vi "Self.vi"(9 "Is Priority":bool, 10 "Msg":refnum<class "Msg.lvclass">, 11 "jettl Actor in":refnum<class "jettl Actor.lvclass">) -> (3 "jettl Actor out":refnum<class "jettl Actor.lvclass">)   [LabVIEW 2021, in "jettl.lvlib" / "Temporary Actor.lvlib" / "jettl Actor.lvclass"]
uses:
  jettl Actor.lvclass
  Msg/Msg.lvclass
  Utilities/Relation.ctl
  jettl Actor.lvclass/jettl Actor.ctl
  Addresses Strategy/Addresses Strategy/Addresses Strategy.lvclass
  Sender/Sender/Sender.lvclass
  Utilities/Utilities.lvlib
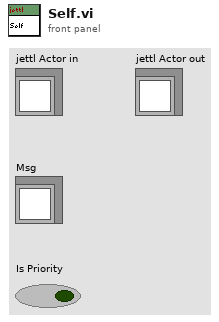
[diagram p1: front panel]
types:
  T1 = typedef "jettl.lvlib/Utilities.lvlib/Relation.ctl" = enum16{"Self", "Creator", "Created"}
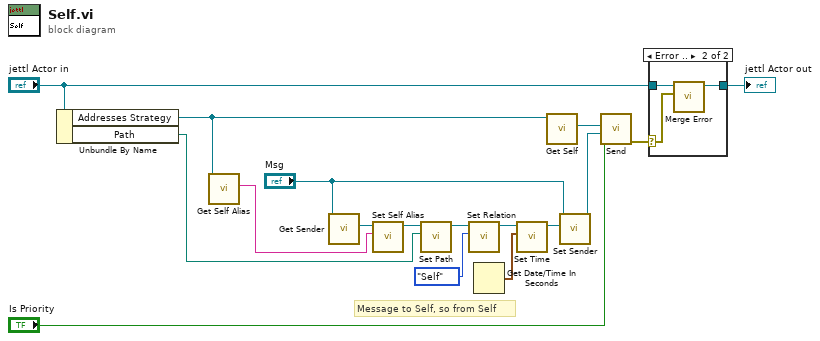
[diagram p0: block diagram]
diagram:
  # "Message to Self, so from Self"
  n1 = Unbundle By Name("jettl Actor in") -> ("Addresses Strategy"=w11:refnum<class "Addresses Strategy.lvclass">, "Path"=w1:path)
  n2 = call-dynamic "Get Self Alias.vi"("Addresses Strategy in"=w11) -> ("Self Alias"=w4:string)  [unwired: 10 in]
  n3 = call-dynamic "Get Sender.vi"("Msg in"="Msg") -> ("Sender"=w6:refnum<class "Sender.lvclass">)  [unwired: 10 in]
  n4 = call-dynamic "Set Self Alias.vi"("Self Alias"=w4, "Sender in"=w6) -> ("Sender out"=w9:refnum<class "Sender.lvclass">)  [unwired: 9 in]
  n5 = call-dynamic "Set Path.vi"("Path"=w1, "Sender in"=w9) -> ("Sender out"=w8:refnum<class "Sender.lvclass">)  [unwired: 9 in]
  n6 = call-dynamic "Set Relation.vi"("Relation"=Relation."Self", "Sender in"=w8) -> ("Sender out"=w7:refnum<class "Sender.lvclass">)  [unwired: 9 in]
  n7 = Get Date/Time In Seconds() -> (seconds since 1Jan1904=w2:timestamp)
  n8 = call-dynamic "Set Time.vi"("Time"=w2, "Sender in"=w7) -> ("Sender out"=w5:refnum<class "Sender.lvclass">)  [unwired: 9 in]
  n9 = call-dynamic "Get Self.vi"("Addresses Strategy in"=w11) -> ("Self"=w15:refnum<user-event>)  [unwired: 10 in]
  n10 = call-dynamic "Set Sender.vi"("Sender"=w5, "Msg in"="Msg") -> ("Msg out"=w12:refnum<class "Msg.lvclass">)  [unwired: 9 in]
  n11 = call "Send.vi"("Is Priority"="Is Priority", "Msg"=w12, "Msg Event"=w15) -> ("error out"=w13:errorcluster)  [unwired: 8 in]
  n12 = case shown="Error .." w13 {
    selector: w13 -> [_ w19]
    tunnel: [w18 w21] -> w16
    tunnel: "jettl Actor in" -> [w18 w20]
    frame No Error {
    }
    frame Error {
      n13 = call-dynamic "Merge Error.vi"("Error"=w19, "jettl Actor in"=w20) -> ("jettl Actor out"=w21:refnum<class "jettl Actor.lvclass">)  [unwired: 9 in]
    }
  }
  "jettl Actor out" <- w16
